vi "exnSpectralBlock clear magnitude.vi"(1 "magnitude in":cluster{"f0":dbl, "df":dbl, "magnitude":dbl[]} {"magnitude" format="%.2p"; "f0" format="%0.2p"; "df" format="%0.2p"}) -> (0 "magnitude out":cluster{"f0":dbl, "df":dbl, "magnitude":dbl[]} {"magnitude" format="%.2p"; "f0" format="%0.2p"; "df" format="%0.2p"})   [LabVIEW 2020]
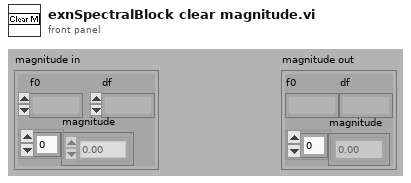
[diagram p1: front panel]
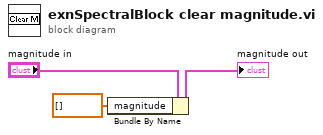
[diagram p0: block diagram]
diagram:
  n1 = Bundle By Name(cluster="magnitude in", "magnitude"=dbl[] []) -> (→"magnitude out":cluster{"f0":dbl, "df":dbl, "magnitude":dbl[]})
